vi "Periodic Tasks.vi"(8 "error in":errorcluster) -> ()   [LabVIEW 2012]
doc: "This VI runs in parallel to other tasks. It can contain as many user-defined periodic loops as you need. These can carry out PID or other sorts of timed response."
uses:
  <vilib>/Rock Robotics/WPI/Relay/WPI_RelayValue.ctl
  <vilib>/Rock Robotics/SystemInterfaces/Utilities/FPGA_UtilitiesLED Source.ctl
  <vilib>/Rock Robotics/SystemInterfaces/Utilities/FPGA_UtilitiesLED State.ctl
  <vilib>/Rock Robotics/WPI/Joystick/WPI_JoystickGetSetRefNum.vi
  Robot Global Data.vi
  <vilib>/Rock Robotics/WPI/Solenoid/WPI_SolenoidSetEnum.vi
  <vilib>/Rock Robotics/WPI/Compressor/WPI_CompressorGetSetRefNum.vi
panel:
  out "Trigger piston":T1
  out "Total Number of shots made":i16
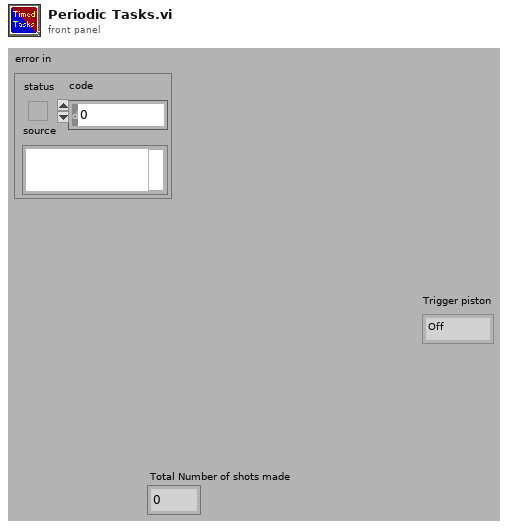
[diagram p1: front panel]
types:
  T1 = typedef "WPI_RelayValue.ctl" = enum16{"Off", "On", "Forward", "Reverse"}
  T2 = typedef "WPI_JoystickDevRef.ctl" = cluster{"Device":T3}
  T3 = typedef "WPI_JoystickDeviceEnum.ctl" = enum16{"USB 1", "USB 2", "USB 3", "USB 4", "Kinect 1", "Kinect 2"}
  T4 = typedef "WPI_EncoderDevRef.ctl" = cluster{"DevStatus":errorcluster, "EncoderIndex":T5, "CounterIndex":T6, "DistancePerCount":dbl, "Decoding Type":T7}
  T5 = typedef "FPGA_EncoderIdx.ctl" = enum8{"Enc 0", "Enc 1", "Enc 2", "Enc 3", "Invalid"}
  T6 = typedef "FPGA_CounterCtrSystemIndex.ctl" = enum8{"Ctr 0", "Ctr 1", "Ctr 2", "Ctr 3", "Ctr 4", "Ctr 5", "Ctr 6", "Ctr 7", "Invalid"}
  T7 = typedef "WPI_EncoderType.ctl" = enum16{"1x", "2x", "4x"}
  T8 = typedef "WPI_DigitalInputDevRef.ctl" = cluster{"DevStatus":errorcluster, "DIO Channel":T9, "Digital Module":T10}
  T9 = typedef "FPGA_DIOChannel.ctl" = enum8{"DIO 1", "DIO 2", "DIO 3", "DIO 4", "DIO 5", "DIO 6", "DIO 7", "DIO 8", "DIO 9", "DIO 10", "DIO 11", "DIO 12", "DIO 13", "DIO 14", "Invalid"}
  T10 = typedef "FPGA_TypedefDigitalModule.ctl" = enum16{"Digital Module 1", "Digital Module 2"}
  T11 = typedef "WPI_MotorControlDeviceRef.ctl" = cluster{"DeviceStatus":errorcluster, "Type":enum16{"PWM", "CAN"}, "PWM":cluster{"Digital Module":T10, "PWM Channel":T12, "DeadBand":T13}, "CAN":cluster{"Device Number":u8, "Control Mode":T14, "Semaphore":T15, "Max Vout":dbl}, "Invert":bool, "TransformRef":T16, "InvTransformRef":T16}
  T12 = typedef "FPGA_DIOPWMChannel.ctl" = enum8{"PWM 1", "PWM 2", "PWM 3", "PWM 4", "PWM 5", "PWM 6", "PWM 7", "PWM 8", "PWM 9", "PWM 10", "Invalid"}
  T13 = typedef "WPI_PWMDeadband.ctl" = cluster{"Name":string, "maxPositivePwm":i32, "minPositivePwm":i32, "centerPwm":i32, "maxNegativePwm":i32, "minNegativePwm":i32, "angularRange":u16}
  T14 = typedef "WPI_CANJaguar_ControlMode.ctl" = enum8{"Percent VBus", "Current", "Speed", "Position", "Voltage"}
  T15 = typedef "Semaphore RefNum" = refnum<k1>
  T16 = typedef "WPI_PWMTransform_ConPane.ctl" = refnum<vi>
  T17 = typedef "WPI_SolenoidDevRef.ctl" = cluster{"DevStatus":errorcluster, "Solenoid Module":T18, "Forward Solenoid Channel":T19, "Reverse Solenoid Channel":T19}
  T18 = typedef "FPGA_TypedefSolenoidModule.ctl" = enum16{"Solenoid Module 1", "Solenoid Module 2"}
  T19 = typedef "WPI_SolenoidChannel.ctl" = enum8{"Solenoid 1", "Solenoid 2", "Solenoid 3", "Solenoid 4", "Solenoid 5", "Solenoid 6", "Solenoid 7", "Solenoid 8", "Invalid"}
  T20 = cluster{"MotorControlDevRef":T11, "MotorControlDevRef":T11, "MotorControlDevRef":T11, "EncoderDevRef":T4}
  T21 = typedef "WPI_JoystickButtonState.ctl" = cluster{"Button 1":bool, "Button 2":bool, "Button 3":bool, "Button 4":bool, "Button 5":bool, "Button 6":bool, "Button 7":bool, "Button 8":bool, "Button 9":bool, "Button 10":bool, "Button 11":bool, "Button 12":bool}
  T22 = cluster{"axis 1 (x)":dbl, "axis 2 (y)":dbl, "axis 3 (throttle)":dbl, "axis 4":dbl, "axis 5":dbl, "axis 6":dbl}
  T23 = typedef "FPGA_UtilitiesLED State.ctl" = enum16{"Off", "On", "Toggle"}
  T24 = typedef "FPGA_UtilitiesLED Source.ctl" = enum16{"User LED", "FPGA LED"}
  T25 = typedef "WPI_CompressorDevRef.ctl" = cluster{"DevStatus":errorcluster, "DigitalInputDevRef":T8, "RelayDevRef":T26}
  T26 = typedef "WPI_RelayDevRef.ctl" = cluster{"DevStatus":errorcluster, "Relay Channel":T27, "Digital Module":T10, "Relay Direction":T28}
  T27 = typedef "FPGA_DIORelayChannel.ctl" = enum8{"Relay 1", "Relay 2", "Relay 3", "Relay 4", "Relay 5", "Relay 6", "Relay 7", "Relay 8", "Invalid"}
  T28 = typedef "WPI_RelayDirection.ctl" = enum16{"Both directions", "Forward only", "Reverse only"}
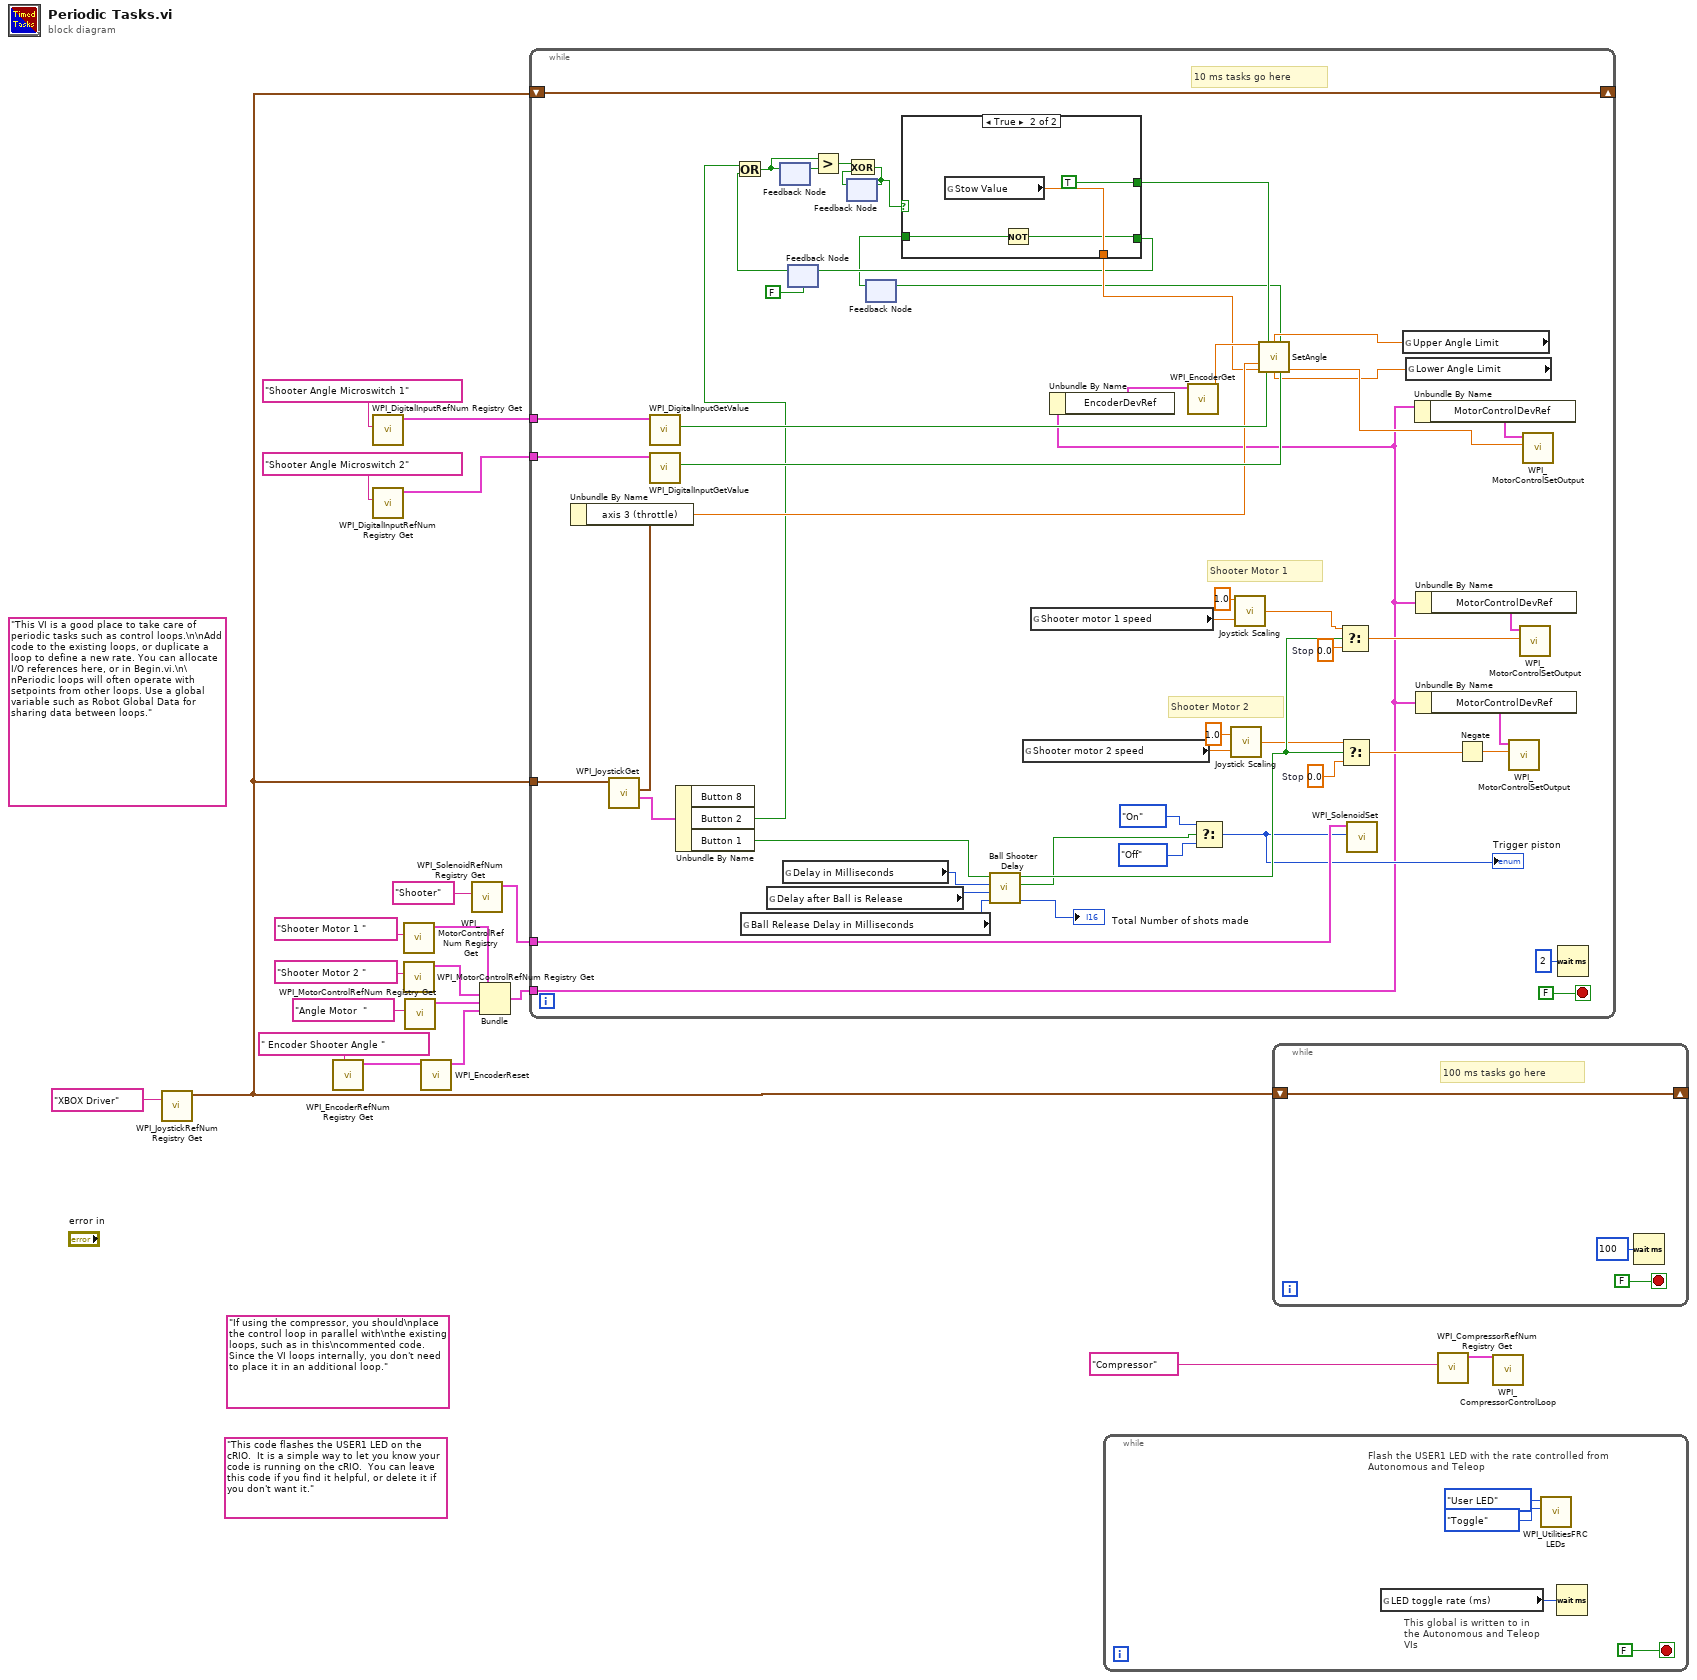
[diagram p0: block diagram]
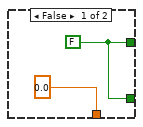
[diagram p2: hidden frame]
diagram:
  (unwired) "If using the compressor, you should\nplace the control loop in parallel with\nthe existing loops, such as in this\ncommented code. Since the VI loops internally, you don't need to place it in an additional loop."
  (unwired) "This code flashes the USER1 LED on the cRIO.  It is a simple way to let you know your code is running on the cRIO.  You can leave this code if you find it helpful, or delete it if you don't want it."
  (unwired) "This VI is a good place to take care of periodic tasks such as control loops.\n\nAdd code to the existing loops, or duplicate a loop to define a new rate. You can allocate I/O references here, or in Begin.vi.\n\nPeriodic loops will often operate with setpoints from other loops. Use a global variable such as Robot Global Data for sharing data between loops."
  n1 = call <vilib>:"WPI_JoystickRefNum Registry Get.vi"("refnum name"="XBOX Driver") -> ("JoystickDevRef"=w11:T2)  [unwired: 1 in, 9 out]
  n2 = call <vilib>:"WPI_EncoderRefNum Registry Get.vi"("refnum name"=" Encoder Shooter Angle ") -> ("EncoderDevRef"=w10:T4)  [unwired: 9 in, 1 out]
  n3 = call <vilib>:"WPI_DigitalInputRefNum Registry Get.vi"("refnum name"="Shooter Angle Microswitch 1") -> ("DigitalInputDevRef"=w7:T8)  [unwired: 9 in, 1 out]
  n4 = call <vilib>:"WPI_DigitalInputRefNum Registry Get.vi"("refnum name"="Shooter Angle Microswitch 2") -> ("DigitalInputDevRef"=w6:T8)  [unwired: 9 in, 1 out]
  n5 = call <vilib>:"WPI_MotorControlRefNum Registry Get.vi"("refnum name"="Shooter Motor 1 ") -> ("MotorControlDevRef"=w18:T11)  [unwired: 9 in, 1 out]
  n6 = call <vilib>:"WPI_MotorControlRefNum Registry Get.vi"("refnum name"="Shooter Motor 2 ") -> ("MotorControlDevRef"=w17:T11)  [unwired: 9 in, 1 out]
  n7 = call <vilib>:"WPI_MotorControlRefNum Registry Get.vi"("refnum name"="Angle Motor  ") -> ("MotorControlDevRef"=w4:T11)  [unwired: 9 in, 1 out]
  n8 = call <vilib>:"WPI_EncoderReset.vi"("EncoderDevRef"=w10) -> ("EncoderDevRef"=w2:T4)  [unwired: 9 in, 1 out]
  n9 = call <vilib>:"WPI_SolenoidRefNum Registry Get.vi"("refnum name"="Shooter") -> ("SolenoidDevRef"=w15:T17)  [unwired: 9 in, 1 out]
  n10 = Bundle("MotorControlDevRef"=w18, "MotorControlDevRef"=w17, "MotorControlDevRef"=w4, "EncoderDevRef"=w2) -> (w14:T20)  [unwired: 1 out]
  n11 = while {
    shift-right: [w73] -> _
    shift-left: w11 -> [w73]
    tunnel: w15 -> [w54]
    tunnel: w14 -> [w26]
    tunnel: w11 -> [w52]
    tunnel: w7 -> [w46]
    tunnel: w6 -> [w45]
    stop <- FALSE stop-if-true
    w62 = 0.0  # Stop
    w69 = 0.0  # Stop
    # "Shooter Motor 1"
    # "Shooter Motor 2"
    # "10 ms tasks go here"
    n12 = call <vilib>:"WPI_JoystickGet.vi"("JoystickDevRef"=w52) -> ("Buttons"=w51:T21, "Axes"=w44:T22)  [unwired: 1 in, 4 out]
    n13 = Unbundle By Name(w44) -> ("axis 3 (throttle)"=w43:dbl)
    n14 = call <vilib>:"WPI_DigitalInputGetValue.vi"("DigitalInputDevRef"=w46) -> ("Value"=w47:bool)  [unwired: 8 in, 2 out]
    n15 = call <vilib>:"WPI_DigitalInputGetValue.vi"("DigitalInputDevRef"=w45) -> ("Value"=w48:bool)  [unwired: 8 in, 2 out]
    n16 = Unbundle By Name(w51) -> ("Button 2"=w36:bool, "Button 1"=w50:bool)  [unwired: 1 out]
    n17 = global read "Robot Global Data.vi" "Ball Release Delay in Milliseconds"() -> (w72:i32)
    n18 = global read "Robot Global Data.vi" "Delay after Ball is Release"() -> (w71:u32)
    n19 = feedback #1() -> (w37:bool)  [unwired: 1 in]
    n20 = global read "Robot Global Data.vi" "Delay in Milliseconds"() -> (w70:i32)
    n21 = feedback #2(FALSE ("Auto Angle")) -> (w34:bool)
    n22 = Or(x=w36, y=w34) -> (x .or. y?=w40:bool)
    n23 = feedback-in #1(w40) -> ()
    n24 = Greater?(x=w40, y=w37) -> (0:w38:bool)
    n25 = feedback #3() -> (w39:bool)  [unwired: 1 in]
    n26 = Exclusive Or(1:w39, 2:w38) -> (0:w35:bool)
    n27 = feedback-in #3(w35) -> ()
    n28 = feedback #4() -> (w21:bool)  [unwired: 1 in]
    n29 = case shown="True" w35 {
      tunnel: [w76 TRUE] -> w42
      tunnel: [0.0 ("Stow Value") w80] -> w41
      tunnel: [w76 w78] -> w23
      tunnel: w21 -> [_ w79]
      frame False {
        w76 = FALSE
      }
      frame True {
        n30 = global read "Robot Global Data.vi" "Stow Value"() -> (w80:dbl)
        n31 = Not(x=w79) -> (.not. x?=w78:bool)
      }
    }
    n32 = feedback-in #2(w23) -> ()
    n33 = call "Ball Shooter Delay.vi"("Ball Release \nDelay in Milliseconds"=w72, "Delay after Ball is Release"=w71, "Delay in Milliseconds"=w70, "Shoot ball"=w50) -> ("Total Number of shots made"=→"Total Number of shots made":i16, "Ball Release"=w53:bool, "Shooter Motor"=w57:bool)  [unwired: 5 in]
    n34 = global read "Robot Global Data.vi" "Shooter motor 2 speed"() -> (w55:dbl)
    n35 = global read "Robot Global Data.vi" "Shooter motor 1 speed"() -> (w56:dbl)
    n36 = Unbundle By Name(w26) -> ("EncoderDevRef"=w25:T4)
    n37 = call <vilib>:"WPI_EncoderGet.vi"("EncoderDevRef"=w25) -> ("Distance"=w49:dbl)  [unwired: 1 in, 9 out]
    n38 = Select(t=WPI_RelayValue."On" ("RelayValue"), s=w53, f=WPI_RelayValue."Off" ("RelayValue")) -> (s? t:f=w31:T1)
    "Trigger piston" <- w31
    n39 = call "Joystick Scaling.vi"("Scale (%)"=w55, "Input (+/- 1.00 volt)"=1.0) -> ("Output"=w27:dbl)  [unwired: 1 in]
    n40 = call "Joystick Scaling.vi"("Scale (%)"=w56, "Input (+/- 1.00 volt)"=1.0) -> ("Output"=w28:dbl)  [unwired: 1 in]
    n41 = Select(t=w28, s=w57, f=w62) -> (s? t:f=w61:dbl)
    n42 = Select(t=w27, s=w57, f=w69) -> (s? t:f=w60:dbl)
    n43 = call-poly <vilib>:"WPI_SolenoidSet.vi"("Value"=w31, "SolenoidDevRef"=w54) -> ()  [unwired: 8 in, 2 out]
    n44 = global read "Robot Global Data.vi" "Upper Angle Limit"() -> (w30:dbl)
    n45 = global read "Robot Global Data.vi" "Lower Angle Limit"() -> (w29:dbl)
    n46 = call "SetAngle.vi"("Encoder distance"=w49, "Camera Enabled"=w42, "encoder upper limit"=w30, "Manual Speed"=w43, "Automatic\nDistance"=w41, "Switch near pivot\n(DIO 3)"=w47, "encoder lower limit"=w29, "Switch near motor\n(DIO 4)"=w48) -> ("Auto Angle"=w22:bool, "Motor Speed"=w33:dbl)  [unwired: 3 in, 3 out]
    n47 = feedback-in #4(w22) -> ()
    n48 = Unbundle By Name(w26) -> ("MotorControlDevRef"=w32:T11)
    n49 = Unbundle By Name(w26) -> ("MotorControlDevRef"=w63:T11)
    n50 = Unbundle By Name(w26) -> ("MotorControlDevRef"=w66:T11)
    n51 = Negate(x=w60) -> (-x=w59:dbl)
    n52 = call <vilib>:"WPI_MotorControlSetOutput.vi"("Output"=w59, "MotorControlDevRef"=w66) -> ()  [unwired: 7 in, 3 out]
    n53 = call <vilib>:"WPI_MotorControlSetOutput.vi"("Output"=w61, "MotorControlDevRef"=w63) -> ()  [unwired: 7 in, 3 out]
    n54 = call <vilib>:"WPI_MotorControlSetOutput.vi"("Output"=w33, "MotorControlDevRef"=w32) -> ()  [unwired: 7 in, 3 out]
    n55 = Wait (ms)(milliseconds to wait=u32 2) -> ()  [unwired: 1 out]
  }
  n56 = while {
    stop <- FALSE stop-if-true
    # "This global is written to in the Autonomous and Teleop VIs"
    # "Flash the USER1 LED with the rate controlled from Autonomous and Teleop"
    n57 = global read "Robot Global Data.vi" "LED toggle rate (ms)"() -> (w82:u32)
    n58 = call <vilib>:"WPI_UtilitiesFRC LEDs.vi"("State"=FPGA_UtilitiesLED_State."Toggle", "LED Type"=FPGA_UtilitiesLED_Source."User LED") -> ()  [unwired: 1 in, 9 out]
    n59 = Wait (ms)(milliseconds to wait=w82) -> ()  [unwired: 1 out]
  }
  n60 = while {
    shift-right: [w86] -> _
    shift-left: w11 -> [w86]
    stop <- FALSE stop-if-true
    # "100 ms tasks go here"
    n61 = Wait (ms)(milliseconds to wait=u32 100) -> ()  [unwired: 1 out]
  }
  n62 = call <vilib>:"WPI_CompressorRefNum Registry Get.vi"("refnum name"="Compressor") -> ("CompressorDevRef"=w20:T25)  [unwired: 9 in, 1 out]
  n63 = call <vilib>:"WPI_CompressorControlLoop.vi"("CompressorDevRef"=w20) -> ()  [unwired: 11 in]
